vi "WriteCommand.vi"(8 "error in (no error)":errorcluster, 11 "StepperMotorController in":refnum<class "StepperMotorController.lvclass">) -> (0 "error out":errorcluster, 3 "StepperMotorController out":refnum<class "StepperMotorController.lvclass">)   [LabVIEW 2023, in "StepperMotorController.lvclass"]
uses:
  StepperMotorController.lvclass
panel:
  in  "Command":string
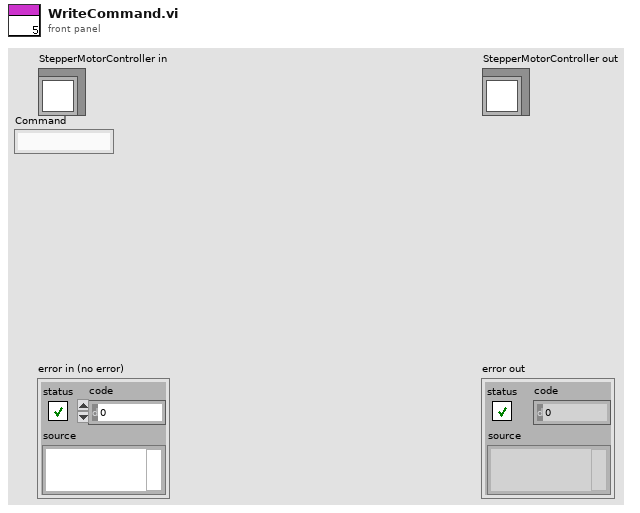
[diagram p1: front panel]
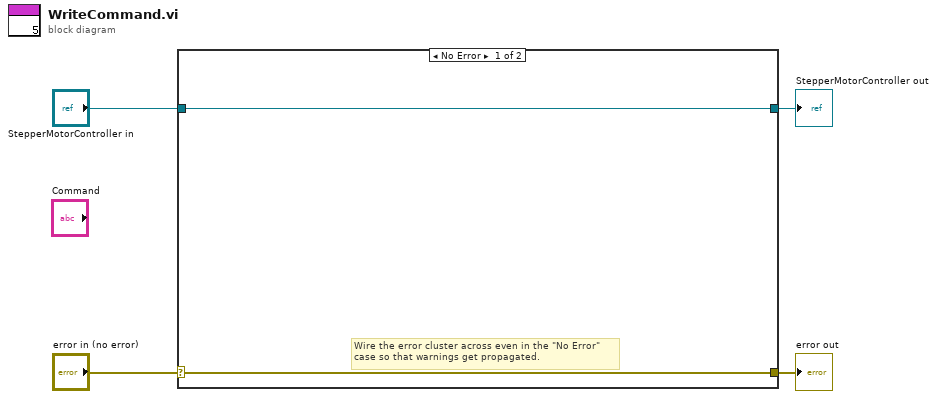
[diagram p0: block diagram]
diagram:
  n1 = case shown="No Error" "error in (no error)" {
    selector: "error in (no error)" -> [w5 w8]
    tunnel: [w5 w8] -> w3
    tunnel: [w6 w7] -> w1
    tunnel: "StepperMotorController in" -> [w6 w7]
    frame No Error {
      # "Wire the error cluster across even in the \"No Error\"\ncase so that warnings get propagated."
    }
    frame Error {
    }
  }
  "error out" <- w3
  "StepperMotorController out" <- w1
